vi "Run.vi"(8 "error in (no error)":errorcluster, 11 "Channel GUI in":refnum<class "Channel GUI.lvclass">) -> (0 "error out":errorcluster, 3 "Channel GUI out":refnum<class "Channel GUI.lvclass">)   [LabVIEW 2018, in "Channel GUI.lvclass"]
uses:
  Channel GUI.lvclass
  Channel GUI.lvclass/Channel GUI.ctl
  State Machine/State Machine.lvclass
  Stream/Stream.lvclass
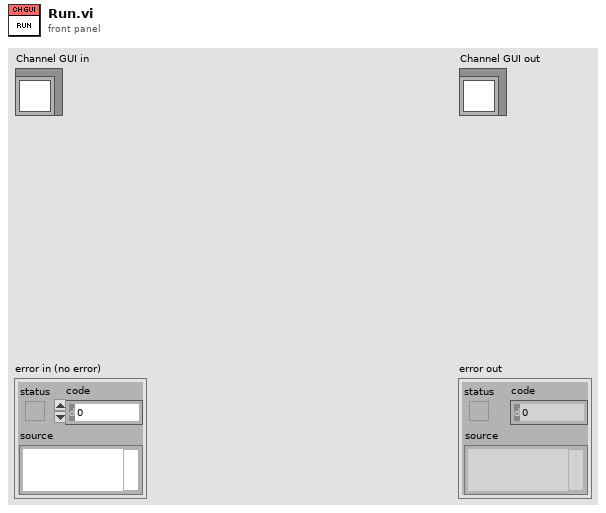
[diagram p1: front panel]
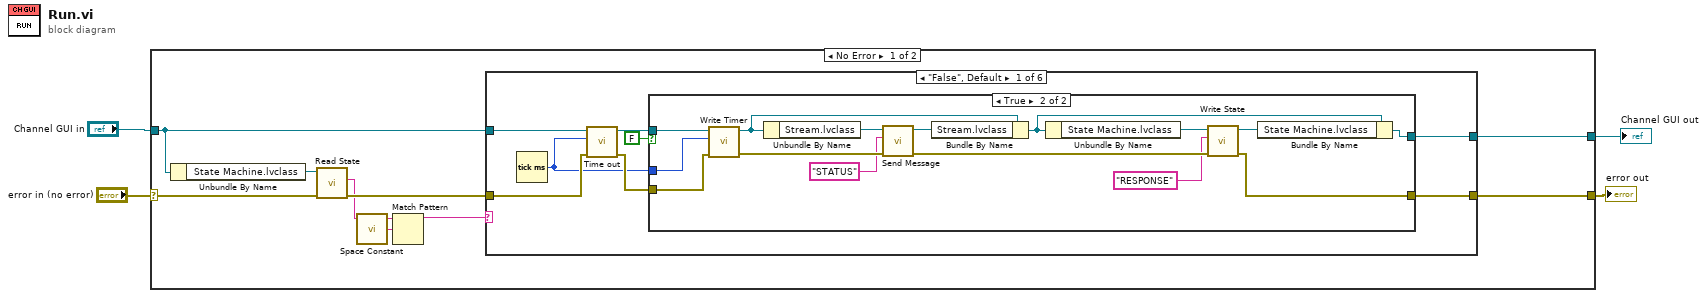
[diagram p0: block diagram]
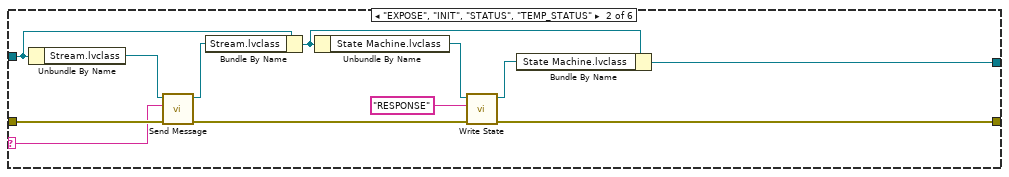
[diagram p3: hidden frame]
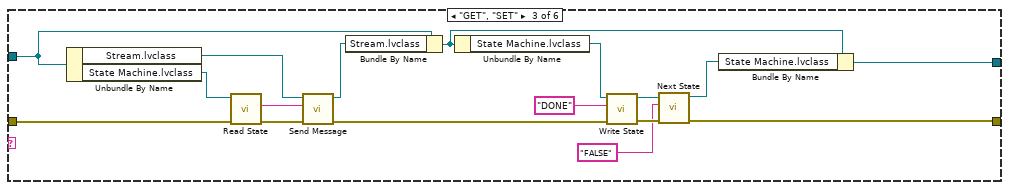
[diagram p4: hidden frame]
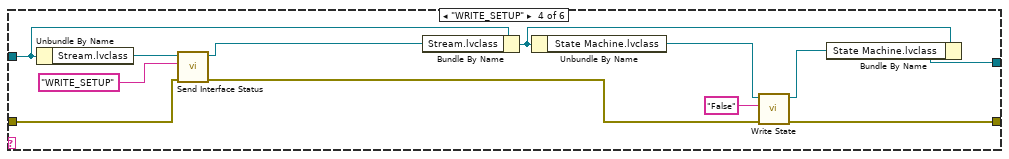
[diagram p5: hidden frame]
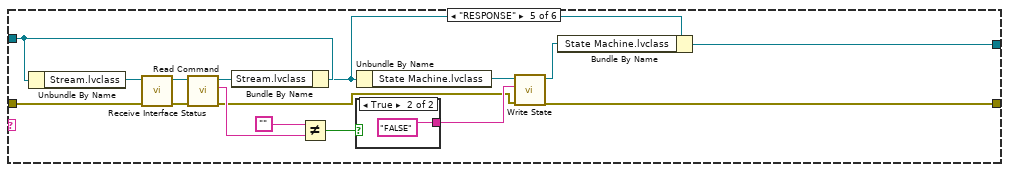
[diagram p6: hidden frame]
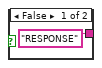
[diagram p7: hidden frame]
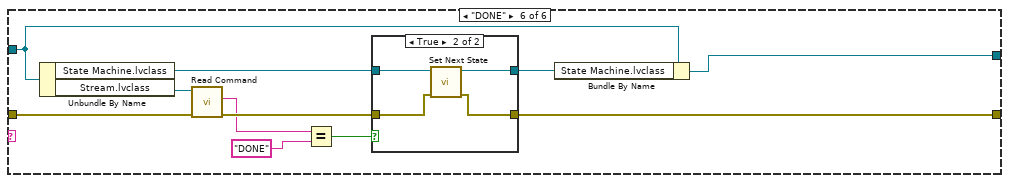
[diagram p8: hidden frame]
diagram:
  n1 = case shown="No Error" "error in (no error)" {
    selector: "error in (no error)" -> [w11 w116]
    tunnel: [w13 w116] -> w2
    tunnel: "Channel GUI in" -> [w9 w115]
    tunnel: [w5 w115] -> w1
    frame No Error {
      n2 = Unbundle By Name(w9) -> ("State Machine.lvclass"=w12:refnum<class "State Machine.lvclass">)
      n3 = call-dynamic "Read State.vi"("error in (no error)"=w11, "State Machine in"=w12) -> ("error out"=w10:errorcluster, "State"=w7:string)  [unwired: 7 in, 1 out]
      n4 = call <vilib>:"Space Constant.vi"() -> ("String"=w8:string)
      n5 = Match Pattern(string=w7, regular expression=w8) -> (before substring=w6:string)  [unwired: 1 in, 3 out]
      n6 = case shown="\"False\", Default" w6 {
        selector: w6 -> [_ w39 _ _ _ _]
        tunnel: w10 -> [w21 w49 w52 w71 w88 w107]
        tunnel: [w17 w42 w56 w75 w94 w99] -> w13
        tunnel: w9 -> [w15 w48 w61 w77 w95 w101]
        tunnel: [w16 w45 w62 w76 w91 w98] -> w5
        frame "False", Default {
          n7 = Tick Count (ms)() -> (millisecond timer value=w18:u32)
          n8 = call "Time out.vi"("error in (no error)"=w21, "New Time"=w18, "Channel GUI in"=w15) -> ("error out"=w19:errorcluster, "Channel GUI out"=w20:refnum<class "Channel GUI.lvclass">)  [unwired: 6 in, 1 out]
          n9 = case shown="True" FALSE {
            tunnel: w20 -> [w23 w27]
            tunnel: w19 -> [w22 w38]
            tunnel: w18 -> [_ w37]
            tunnel: [w22 w30] -> w17
            tunnel: [w23 w28] -> w16
            frame False {
            }
            frame True {
              n10 = call "Write Timer.vi"("error in (no error)"=w38, "Timer"=w37, "Channel GUI in"=w27) -> ("error out"=w35:errorcluster, "Channel GUI out"=w25:refnum<class "Channel GUI.lvclass">)  [unwired: 7 in]
              n11 = Unbundle By Name(w25) -> ("Stream.lvclass"=w26:refnum<class "Stream.lvclass">)
              n12 = call "Send Message.vi"("error in (no error)"=w35, "Message"="STATUS" ("New_State"), "Stream in"=w26) -> ("error out"=w33:errorcluster, "Stream out"=w36:refnum<class "Stream.lvclass">)  [unwired: 7 in]
              n13 = Bundle By Name(cluster=w25, "Stream.lvclass"=w36) -> (w31:refnum<class "Channel GUI.lvclass">)
              n14 = Unbundle By Name(w31) -> ("State Machine.lvclass"=w24:refnum<class "State Machine.lvclass">)
              n15 = call-dynamic "Write State.vi"("error in (no error)"=w33, "State"="RESPONSE" ("New_State"), "State Machine in"=w24) -> ("error out"=w30:errorcluster, "State Machine out"=w32:refnum<class "State Machine.lvclass">)  [unwired: 7 in]
              n16 = Bundle By Name(cluster=w31, "State Machine.lvclass"=w32) -> (w28:refnum<class "Channel GUI.lvclass">)
            }
          }
        }
        frame "EXPOSE", "INIT", "STATUS", "TEMP_STATUS" {
          n17 = Unbundle By Name(w48) -> ("Stream.lvclass"=w50:refnum<class "Stream.lvclass">)
          n18 = call "Send Message.vi"("error in (no error)"=w49, "Message"=w39, "Stream in"=w50) -> ("error out"=w41:errorcluster, "Stream out"=w47:refnum<class "Stream.lvclass">)  [unwired: 7 in]
          n19 = Bundle By Name(cluster=w48, "Stream.lvclass"=w47) -> (w46:refnum<class "Channel GUI.lvclass">)
          n20 = Unbundle By Name(w46) -> ("State Machine.lvclass"=w44:refnum<class "State Machine.lvclass">)
          n21 = call-dynamic "Write State.vi"("error in (no error)"=w41, "State"="RESPONSE" ("New_State"), "State Machine in"=w44) -> ("error out"=w42:errorcluster, "State Machine out"=w43:refnum<class "State Machine.lvclass">)  [unwired: 7 in]
          n22 = Bundle By Name(cluster=w46, "State Machine.lvclass"=w43) -> (w45:refnum<class "Channel GUI.lvclass">)
        }
        frame "GET", "SET" {
          n23 = Unbundle By Name(w61) -> ("Stream.lvclass"=w64:refnum<class "Stream.lvclass">, "State Machine.lvclass"=w54:refnum<class "State Machine.lvclass">)
          n24 = call-dynamic "Read State.vi"("error in (no error)"=w52, "State Machine in"=w54) -> ("error out"=w53:errorcluster, "State"=w51:string)  [unwired: 7 in, 1 out]
          n25 = call "Send Message.vi"("error in (no error)"=w53, "Message"=w51, "Stream in"=w64) -> ("error out"=w67:errorcluster, "Stream out"=w65:refnum<class "Stream.lvclass">)  [unwired: 7 in]
          n26 = Bundle By Name(cluster=w61, "Stream.lvclass"=w65) -> (w66:refnum<class "Channel GUI.lvclass">)
          n27 = Unbundle By Name(w66) -> ("State Machine.lvclass"=w60:refnum<class "State Machine.lvclass">)
          n28 = call-dynamic "Write State.vi"("error in (no error)"=w67, "State"="DONE" ("New_State"), "State Machine in"=w60) -> ("error out"=w59:errorcluster, "State Machine out"=w58:refnum<class "State Machine.lvclass">)  [unwired: 7 in]
          n29 = call "Next State.vi"("error in (no error)"=w59, "New_State"="FALSE", "State Machine in"=w58) -> ("error out"=w56:errorcluster, "State Machine out"=w57:refnum<class "State Machine.lvclass">)  [unwired: 7 in]
          n30 = Bundle By Name(cluster=w66, "State Machine.lvclass"=w57) -> (w62:refnum<class "Channel GUI.lvclass">)
        }
        frame "WRITE_SETUP" {
          n31 = Unbundle By Name(w77) -> ("Stream.lvclass"=w72:refnum<class "Stream.lvclass">)
          n32 = call "Send Interface Status.vi"("error in (no error)"=w71, "Message"="WRITE_SETUP" ("New_State"), "Stream in"=w72) -> ("error out"=w68:errorcluster, "Stream out"=w69:refnum<class "Stream.lvclass">)  [unwired: 7 in]
          n33 = Bundle By Name(cluster=w77, "Stream.lvclass"=w69) -> (w78:refnum<class "Channel GUI.lvclass">)
          n34 = Unbundle By Name(w78) -> ("State Machine.lvclass"=w79:refnum<class "State Machine.lvclass">)
          n35 = call-dynamic "Write State.vi"("error in (no error)"=w68, "State"="False" ("New_State"), "State Machine in"=w79) -> ("error out"=w75:errorcluster, "State Machine out"=w74:refnum<class "State Machine.lvclass">)  [unwired: 7 in]
          n36 = Bundle By Name(cluster=w78, "State Machine.lvclass"=w74) -> (w76:refnum<class "Channel GUI.lvclass">)
        }
        frame "RESPONSE" {
          n37 = Unbundle By Name(w95) -> ("Stream.lvclass"=w89:refnum<class "Stream.lvclass">)
          n38 = call "Receive Interface Status.vi"("error in (no error)"=w88, "Stream in"=w89) -> ("error out"=w87:errorcluster, "Stream out"=w86:refnum<class "Stream.lvclass">)  [unwired: 8 in]
          n39 = call "Read Command.vi"("error in (no error)"=w87, "Stream in"=w86) -> ("error out"=w80:errorcluster, "Command"=w85:string, "Stream out"=w82:refnum<class "Stream.lvclass">)  [unwired: 7 in]
          n40 = Bundle By Name(cluster=w95, "Stream.lvclass"=w82) -> (w92:refnum<class "Channel GUI.lvclass">)
          n41 = Not Equal?(x="", y=w85) -> (x != y?=w83:bool)
          n42 = case shown="True" w83 {
            tunnel: ["RESPONSE" "FALSE"] -> w81
            frame False {
            }
            frame True {
            }
          }
          n43 = Unbundle By Name(w92) -> ("State Machine.lvclass"=w93:refnum<class "State Machine.lvclass">)
          n44 = call-dynamic "Write State.vi"("error in (no error)"=w80, "State"=w81, "State Machine in"=w93) -> ("error out"=w94:errorcluster, "State Machine out"=w90:refnum<class "State Machine.lvclass">)  [unwired: 7 in]
          n45 = Bundle By Name(cluster=w92, "State Machine.lvclass"=w90) -> (w91:refnum<class "Channel GUI.lvclass">)
        }
        frame "DONE" {
          n46 = Unbundle By Name(w101) -> ("State Machine.lvclass"=w102:refnum<class "State Machine.lvclass">, "Stream.lvclass"=w108:refnum<class "Stream.lvclass">)
          n47 = call "Read Command.vi"("error in (no error)"=w107, "Stream in"=w108) -> ("error out"=w106:errorcluster, "Command"=w103:string)  [unwired: 7 in, 1 out]
          n48 = Equal?(x=w103, y="DONE") -> (x = y?=w105:bool)
          n49 = case shown="True" w105 {
            tunnel: [w110 w111] -> w99
            tunnel: w106 -> [w110 w112]
            tunnel: w102 -> [w109 w114]
            tunnel: [w109 w113] -> w100
            frame False {
            }
            frame True {
              n50 = call "Set Next State.vi"("error in (no error)"=w112, "State Machine in"=w114) -> ("error out"=w111:errorcluster, "State Machine out"=w113:refnum<class "State Machine.lvclass">)  [unwired: 8 in]
            }
          }
          n51 = Bundle By Name(cluster=w101, "State Machine.lvclass"=w100) -> (w98:refnum<class "Channel GUI.lvclass">)
        }
      }
    }
    frame Error {
    }
  }
  "error out" <- w2
  "Channel GUI out" <- w1
